vi "Tank to Arcade.vi"(0 "Joystick 2y":dbl, 1 "DriveRefNum":string, 7 "Joystick 1y":dbl, 11 "Joysticl 1z":dbl, 12 "Tank to Arcade":bool, 13 "Invert Control":bool) -> ()   [LabVIEW 2015]
uses:
  <vilib>/Rock Robotics/WPI/Utilities/WPI_GetSetVariantRefNum.vi
  <vilib>/Rock Robotics/WPI/RobotDrive/WPI_RobotDriveArcadeDrive_Standard(NoSaturation).vi
  <vilib>/Rock Robotics/Network Tables/NT Write Numeric Array.vi
  <vilib>/Rock Robotics/Network Tables/NT Write Boolean.vi
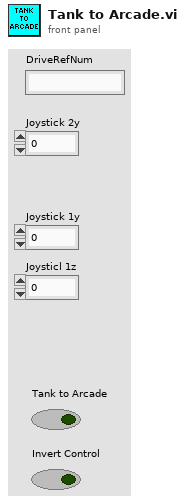
[diagram p1: front panel]
types:
  T1 = typedef "WPI_RobotDriveDevRef.ctl" = cluster{"DevStatus":errorcluster, "Motors[]":T2[], "Square Inputs":bool, "Max Output":dbl}
  T2 = typedef "WPI_MotorControlDeviceRef.ctl" = cluster{"DeviceStatus":errorcluster, "Type":T3, "PWM":cluster{"PWM Channel":T4, "DeadBand":T5}, "CAN":cluster{"Device Number":u8, "Control Mode":T6, "Semaphore":T7, "Max Vout":dbl, "TalonSRX Control Mode":T8}, "Invert":bool}
  T3 = typedef "WPI_MotorControlType.ctl" = enum16{"PWM", "CAN", "CANTalonSRX"}
  T4 = typedef "FPGA_DIOPWMChannel.ctl" = enum8{"PWM 0", "PWM 1", "PWM 2", "PWM 3", "PWM 4", "PWM 5", "PWM 6", "PWM 7", "PWM 8", "PWM 9", "PWM MXP 0", "PWM MXP 1", "PWM MXP 2", "PWM MXP 3", "PWM MXP 4", "PWM MXP 5", "PWM MXP 6", "PWM MXP 7", "PWM MXP 8", "PWM MXP 9", "Invalid"}
  T5 = typedef "WPI_PWMDeadband.ctl" = cluster{"Name":string, "maxPositivePwm":i32, "minPositivePwm":i32, "centerPwm":i32, "maxNegativePwm":i32, "minNegativePwm":i32, "angularRange":u16}
  T6 = typedef "WPI_CANJaguar_ControlMode.ctl" = enum8{"Percent VBus", "Current", "Speed", "Position", "Voltage"}
  T7 = typedef "Semaphore RefNum" = refnum<k1>
  T8 = typedef "WPI_CANTalonSRX_APIControlMode.ctl" = enum8{"Percent VBus", "Speed", "Position", "Slave", "Unchanged / Invalid", "Voltage Compensation", "Current", "Motion Profile"}
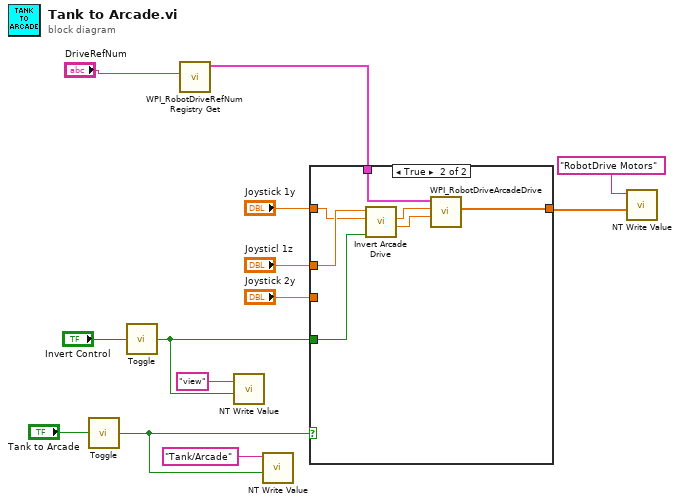
[diagram p0: block diagram]
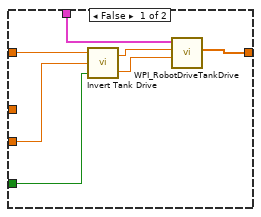
[diagram p2: hidden frame]
diagram:
  n1 = call "Toggle.vi"("Input"="Tank to Arcade") -> ("Output"=w5:bool)
  n2 = call "Toggle.vi"("Input"="Invert Control") -> ("Output"=w1:bool)
  n3 = call <vilib>:"WPI_RobotDriveRefNum Registry Get.vi"("refnum name"="DriveRefNum") -> ("RobotDriveDevRef"=w9:T1)  [unwired: 9 in, 1 out]
  n4 = call-poly <vilib>:"NT Write Value.vi"("Boolean"=w1, "Name"="view") -> ()  [unwired: 9 in, 1 out]
  n5 = call-poly <vilib>:"NT Write Value.vi"("Boolean"=w5, "Name"="Tank/Arcade") -> ()  [unwired: 9 in, 1 out]
  n6 = case shown="True" w5 {
    tunnel: [w20 w27] -> w7
    tunnel: w9 -> [w19 w26]
    tunnel: "Joystick 1y" -> [w18 w22]
    tunnel: "Joystick 2y" -> [w17 _]
    tunnel: "Joysticl 1z" -> [_ w23]
    tunnel: w1 -> [w14 w21]
    frame False {
      n7 = call "Invert Tank Drive.vi"("Toggle"=w14, "Value 2"=w17, "Value 1"=w18) -> ("Value 2"=w15:dbl, "Value 1"=w16:dbl)
      n8 = call <vilib>:"WPI_RobotDriveTankDrive.vi"("Right axis value"=w15, "Left axis value"=w16, "RobotDriveDevRef"=w19) -> ("Motor Values"=w20:dbl[])  [unwired: 6 in, 2 out]
    }
    frame True {
      n9 = call "Invert Arcade Drive.vi"("Toggle"=w21, "Value 2"=w22, "Value 1"=w23) -> ("Value 2"=w24:dbl, "Value 1"=w25:dbl)  [unwired: 7 in]
      n10 = call-poly <vilib>:"WPI_RobotDriveArcadeDrive.vi"("Y axis value"=w24, "X axis value"=w25, "RobotDriveDevRef"=w26) -> ("Motor Values"=w27:dbl[])  [unwired: 6 in, 2 out]
    }
  }
  n11 = call-poly <vilib>:"NT Write Value.vi"("Numeric Array"=w7, "Name"="RobotDrive Motors") -> ()  [unwired: 9 in, 1 out]
